vi "Main.vi"() -> ()   [LabVIEW 2014]
panel:
  in  "Listbox 3":i32(listbox)
  in  "Listbox 2":i32(listbox)
  in  "Listbox":i32(listbox)
  in  "Combo Box":string(combo)
  in  "Numeric":dbl
  in  "Boolean":bool
  in  "stop":bool
  in  "Tree":string(tree)
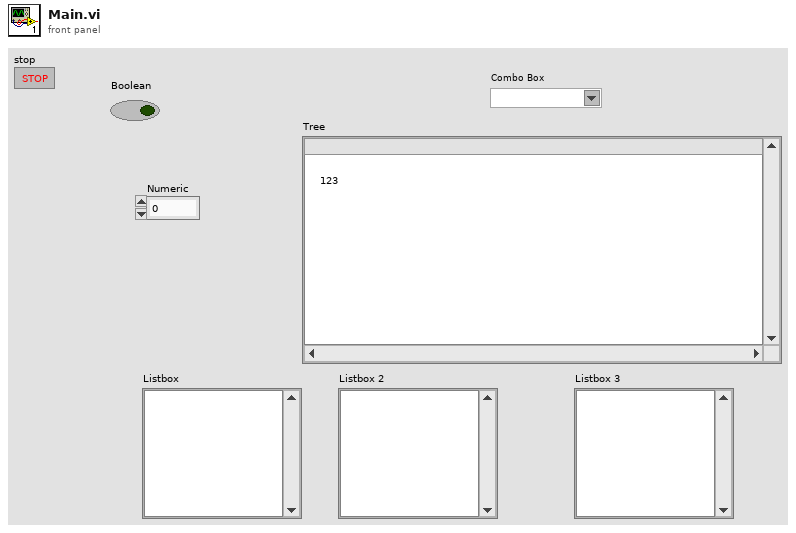
[diagram p1: front panel]
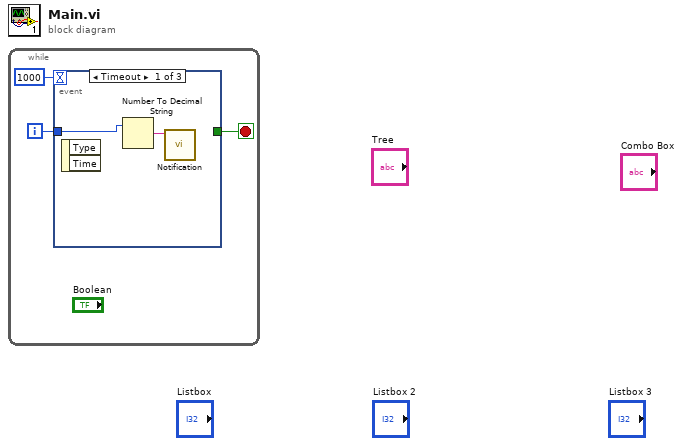
[diagram p0: block diagram]
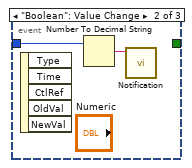
[diagram p2: hidden frame]
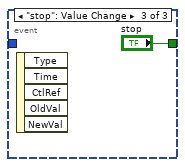
[diagram p3: hidden frame]
diagram:
  n1 = while {
    i -> [w2]
    stop <- w3 stop-if-true
    n2 = event shown="[0] Timeout" {
      selector: _ -> [_ _ _]
      dyn-events: _ -> [_ _ _]
      timeout: 1000 -> [_ _ _]
      tunnel: [_ _ "stop"] -> w3
      tunnel: w2 -> [w4 w7 _]
      event Timeout {
        n3 = event-data() -> ()  [unwired: 1 in, 2 out]
        n4 = Number To Decimal String(number=w4) -> (decimal integer string=w5:string)  [unwired: 1 in]
        n5 = call "Notification.vi"("NotificationBarString"=w5) -> ()  [unwired: 10 in, 1 out]
      }
      event "Boolean": Value Change {
        n6 = event-data() -> ()  [unwired: 1 in, 5 out]
        n7 = Number To Decimal String(number=w7) -> (decimal integer string=w6:string)  [unwired: 1 in]
        n8 = call "Notification.vi"("NotificationBarString"=w6) -> ()  [unwired: 10 in, 1 out]
      }
      event "stop": Value Change {
        n9 = event-data() -> ()  [unwired: 1 in, 5 out]
      }
    }
  }
